vi "TransIntoRequiredFormat(SubVI).vi"(1 "Boolean":bool, 2 "String In":string) -> (0 "String Out":string)   [LabVIEW 2018]
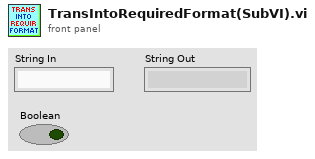
[diagram p1: front panel]
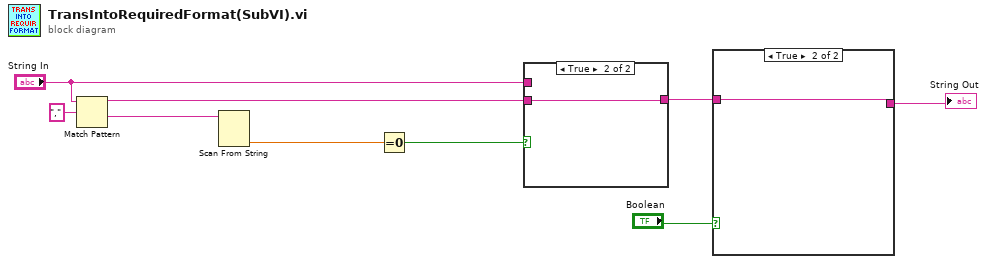
[diagram p0: block diagram]
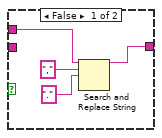
[diagram p2: hidden frame]
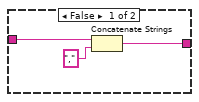
[diagram p3: hidden frame]
diagram:
  n1 = Match Pattern(string="String In", regular expression=",") -> (before substring=w9:string, after substring=w3:string)  [unwired: 1 in, 2 out]
  n2 = Scan From String(input string=w3) -> (output 1=w2:dbl)  [unwired: 4 in, 3 out]
  n3 = Equal To 0?(x=w2) -> (x = 0?=w1:bool)
  n4 = case shown="True" w1 {
    tunnel: w9 -> [_ w14]
    tunnel: [w10 w14] -> w5
    tunnel: "String In" -> [w11 _]
    frame False {
      n5 = Search and Replace String(input string=w11, search string=",", replace string="." ("replace string (\"\")")) -> (result string=w10:string)  [unwired: 5 in, 3 out]
    }
    frame True {
    }
  }
  n6 = case shown="True" "Boolean" {
    tunnel: w5 -> [w16 w18]
    tunnel: [w15 w18] -> w6
    frame False {
      n7 = Concatenate Strings(w16, "," ("string")) -> (w15:string)
    }
    frame True {
    }
  }
  "String Out" <- w6
